vi "start async worker.vi"(8 "error in":errorcluster, 10 "run flag":u8 format="%.0b", 11 "module data in":T1={"run state"=enum."sync", "module"=refnum, "module ref"=refnum, "async exec ref"={"command fifo"=refnum, "error fifo"=refnum, "VI Refnum"=refnum, "input buffer"=refnum, "output buffer"=refnum, "process buffer"=refnum, "original dvrs"=[]}, "configuration ref"=refnum, "GUID"={"Hi"=0, "Lo"=0}, "error"={"status"=FALSE, "code"=0, "source"=""}, "previous error code"=0, "input method"={"data table"={"Double"=[], "Single"=[], "I64"=[], "I32"=[], "I16"=[], "I8"=[], "U64"=[], "U32"=[], "U16"=[], "U8"=[], "Boolean"=[], "String"=[], "Array of Double"=[], "Array of Single"=[], "Array of I64"=[], "Array of I32"=[], "Array of I16"=[], "Array of I8"=[], "Array of U64"=[], "Array of U32"=[], "Array of U16"=[], "Array of U8"=[], "Array of Boolean"=[], "Array of String"=[]}, "transfer spec"=[]}, "output method"={"data table"={"Double"=[], "Single"=[], "I64"=[], "I32"=[], "I16"=[], "I8"=[], "U64"=[], "U32"=[], "U16"=[], "U8"=[], "Boolean"=[], "String"=[], "Array of Double"=[], "Array of Single"=[], "Array of I64"=[], "Array of I32"=[], "Array of I16"=[], "Array of I8"=[], "Array of U64"=[], "Array of U32"=[], "Array of U16"=[], "Array of U8"=[], "Array of Boolean"=[], "Array of String"=[]}, "transfer spec"=[]}, "process method parameters"={"data table"={"Double"=[], "Single"=[], "I64"=[], "I32"=[], "I16"=[], "I8"=[], "U64"=[], "U32"=[], "U16"=[], "U8"=[], "Boolean"=[], "String"=[], "Array of Double"=[], "Array of Single"=[], "Array of I64"=[], "Array of I32"=[], "Array of I16"=[], "Array of I8"=[], "Array of U64"=[], "Array of U32"=[], "Array of U16"=[], "Array of U8"=[], "Array of Boolean"=[], "Array of String"=[]}, "transfer spec"=[]}, "process method results"={"data table"={"Double"=[], "Single"=[], "I64"=[], "I32"=[], "I16"=[], "I8"=[], "U64"=[], "U32"=[], "U16"=[], "U8"=[], "Boolean"=[], "String"=[], "Array of Double"=[], "Array of Single"=[], "Array of I64"=[], "Array of I32"=[], "Array of I16"=[], "Array of I8"=[], "Array of U64"=[], "Array of U32"=[], "Array of U16"=[], "Array of U8"=[], "Array of Boolean"=[], "Array of String"=[]}, "transfer spec"=[]}, "fault handling"={"unknown"=[], "trivial"=[], "critical"=[], "recoverable"=[]}, "error report index "=-1} {"GUID"."Lo" format="%.0x"; "GUID"."Hi" format="%.0x"}) -> (0 "error out":errorcluster, 3 "module data out":T1={"run state"=enum."sync", "module"=refnum, "module ref"=refnum, "async exec ref"={"command fifo"=refnum, "error fifo"=refnum, "VI Refnum"=refnum, "input buffer"=refnum, "output buffer"=refnum, "process buffer"=refnum, "original dvrs"=[]}, "configuration ref"=refnum, "GUID"={"Hi"=0, "Lo"=0}, "error"={"status"=FALSE, "code"=0, "source"=""}, "previous error code"=0, "input method"={"data table"={"Double"=[], "Single"=[], "I64"=[], "I32"=[], "I16"=[], "I8"=[], "U64"=[], "U32"=[], "U16"=[], "U8"=[], "Boolean"=[], "String"=[], "Array of Double"=[], "Array of Single"=[], "Array of I64"=[], "Array of I32"=[], "Array of I16"=[], "Array of I8"=[], "Array of U64"=[], "Array of U32"=[], "Array of U16"=[], "Array of U8"=[], "Array of Boolean"=[], "Array of String"=[]}, "transfer spec"=[]}, "output method"={"data table"={"Double"=[], "Single"=[], "I64"=[], "I32"=[], "I16"=[], "I8"=[], "U64"=[], "U32"=[], "U16"=[], "U8"=[], "Boolean"=[], "String"=[], "Array of Double"=[], "Array of Single"=[], "Array of I64"=[], "Array of I32"=[], "Array of I16"=[], "Array of I8"=[], "Array of U64"=[], "Array of U32"=[], "Array of U16"=[], "Array of U8"=[], "Array of Boolean"=[], "Array of String"=[]}, "transfer spec"=[]}, "process method parameters"={"data table"={"Double"=[], "Single"=[], "I64"=[], "I32"=[], "I16"=[], "I8"=[], "U64"=[], "U32"=[], "U16"=[], "U8"=[], "Boolean"=[], "String"=[], "Array of Double"=[], "Array of Single"=[], "Array of I64"=[], "Array of I32"=[], "Array of I16"=[], "Array of I8"=[], "Array of U64"=[], "Array of U32"=[], "Array of U16"=[], "Array of U8"=[], "Array of Boolean"=[], "Array of String"=[]}, "transfer spec"=[]}, "process method results"={"data table"={"Double"=[], "Single"=[], "I64"=[], "I32"=[], "I16"=[], "I8"=[], "U64"=[], "U32"=[], "U16"=[], "U8"=[], "Boolean"=[], "String"=[], "Array of Double"=[], "Array of Single"=[], "Array of I64"=[], "Array of I32"=[], "Array of I16"=[], "Array of I8"=[], "Array of U64"=[], "Array of U32"=[], "Array of U16"=[], "Array of U8"=[], "Array of Boolean"=[], "Array of String"=[]}, "transfer spec"=[]}, "fault handling"={"unknown"=[], "trivial"=[], "critical"=[], "recoverable"=[]}, "error report index "=-1} {"GUID"."Lo" format="%.0x"; "GUID"."Hi" format="%.0x"})   [LabVIEW 2013, in "async executor.lvlib"]
uses:
  async executor.lvlib
  Runtime/full module data.ctl
  <vilib>/NI/Tag Bus Module Framework/runtime/TBM module execution interface.lvclass
  Runtime/module run state.ctl
  asynchronous executor reference.ctl
  message to executor.ctl
  Runtime/async command notification.ctl
  <vilib>/NI/Tag Bus/table/data table.ctl
  Runtime/async error info.ctl
  <vilib>/NI/Tag Bus Module Framework/runtime/error classification.ctl
  <vilib>/NI/Tag Bus Module Framework/module configuration/TBM module configuration.lvclass
  <vilib>/NI/Configuration Framework/serializable configuration/Numeric GUID.ctl
  Runtime/module method data.ctl
  <vilib>/NI/Tag Bus/table/transfer specification.ctl
  <vilib>/NI/Tag Bus/tag/Data Type.ctl
  Runtime/fault handling spec.ctl
  Configuration/Error Actions.ctl
  async worker process.vi
  <vilib>/NI/Tag Bus/table/data table.lvlib
  main engine/main engine.lvlib
  <vilib>/NI/Tag Bus/tag/tag descriptor.lvclass
  Configuration/Standard Engine Configuration.lvclass
  <vilib>/NI/Configuration Framework/serializable configuration/NISE_CEF_serializable configuration.lvclass
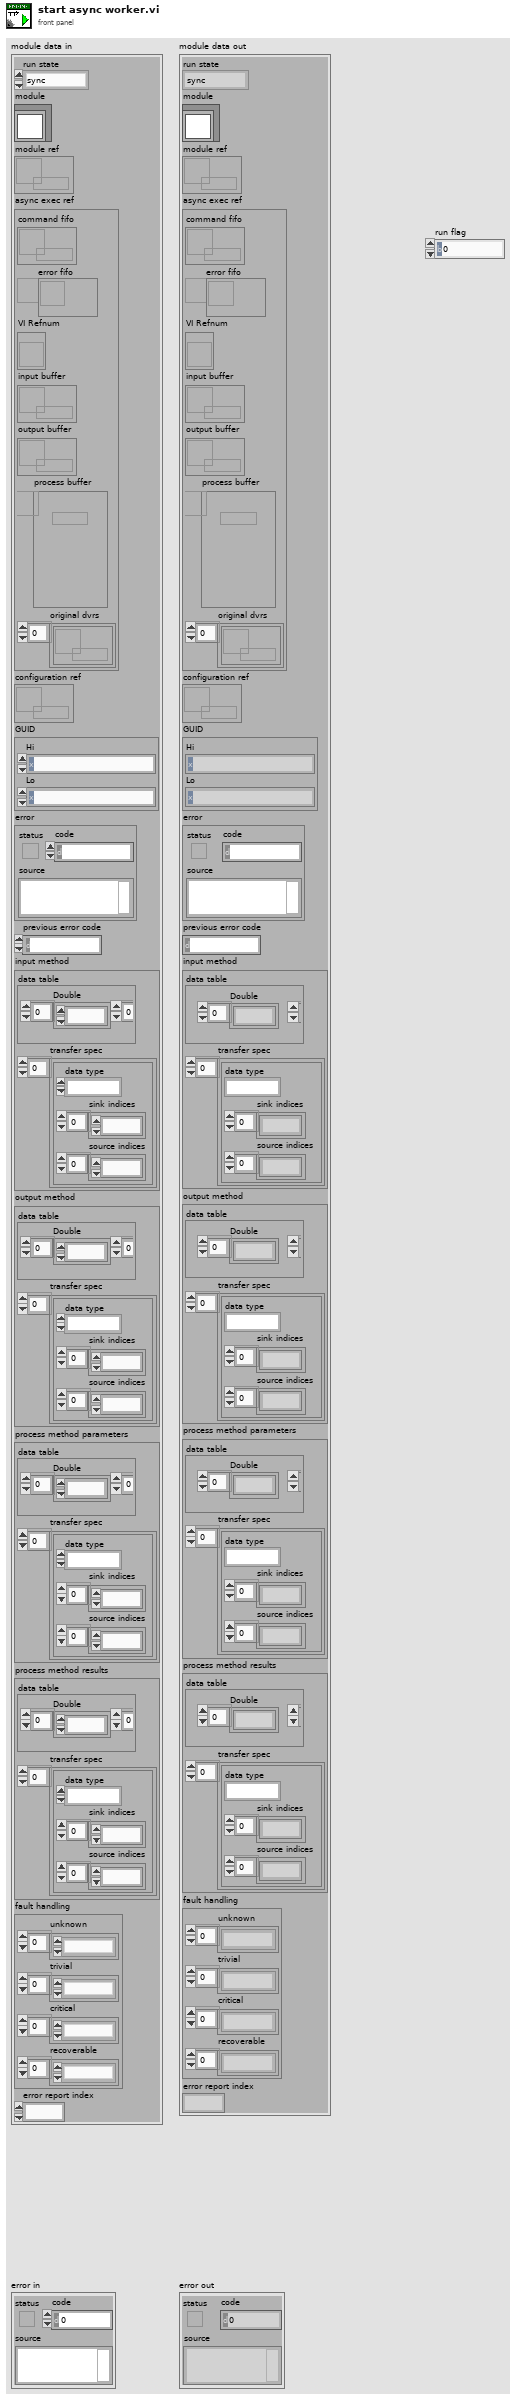
[diagram p1: front panel]
types:
  T1 = typedef "main engine.lvlib/full module data.ctl" = cluster{"run state":T2, "module":refnum<class "TBM module execution interface.lvclass">, "module ref":refnum<data-value>, "async exec ref":T3, "configuration ref":refnum<data-value>, "GUID":T4, "error":errorcluster, "previous error code":i32, "input method":T5, "output method":T5, "process method parameters":T5, "process method results":T5, "fault handling":T9, "error report index ":i32}
  T2 = typedef "main engine.lvlib/module run state.ctl" = enum16{"sync", "async"}
  T3 = typedef "async executor.lvlib/asynchronous executor reference.ctl" = cluster{"command fifo":refnum<k33>, "error fifo":refnum<k33>, "VI Refnum":refnum<vi>, "input buffer":refnum<k33>, "output buffer":refnum<k33>, "process buffer":refnum<k33>, "original dvrs":refnum<data-value>[]}
  T4 = typedef "NISE_CEF_serializable configuration.lvclass/Numeric GUID.ctl" = cluster{"Hi":u64, "Lo":u64}
  T5 = typedef "main engine.lvlib/module method data.ctl" = cluster{"data table":T6, "transfer spec":T7[]}
  T6 = typedef "tag bus.lvlib/data table.lvlib/data table.ctl" = cluster{"Double":dbl[], "Single":sgl[], "I64":i64[], "I32":i32[], "I16":i16[], "I8":i8[], "U64":u64[], "U32":u32[], "U16":u16[], "U8":u8[], "Boolean":bool[], "String":string[], "Array of Double":cluster{"DBL Array":dbl[]}[], "Array of Single":cluster{"SGL Array":sgl[]}[], "Array of I64":cluster{"I64 Array":i64[]}[], "Array of I32":cluster{"I32 Array":i32[]}[], "Array of I16":cluster{"I16 Array":i16[]}[], "Array of I8":cluster{"I8 Array":i8[]}[], "Array of U64":cluster{"U64 Array":u64[]}[], "Array of U32":cluster{"U32 Array":u32[]}[], "Array of U16":cluster{"U16 Array":u16[]}[], "Array of U8":cluster{"U8 Array":u8[]}[], "Array of Boolean":cluster{"Boolean Array":bool[]}[], "Array of String":cluster{"String Array":string[]}[]}
  T7 = typedef "tag bus.lvlib/data table.lvlib/transfer specification.ctl" = cluster{"data type":T8, "sink indices":i32[], "source indices":i32[]}
  T8 = typedef "tag bus.lvlib/tag descriptor.lvclass/Data Type.ctl" = enum16{"Double", "Single", "I64", "I32", "I16", "I8", "U64", "U32", "U16", "U8", "Boolean", "String", "Array of Double", "Array of Single", "Array of I64", "Array of I32", "Array of I16", "Array of I8", "Array of U64", "Array of U32", "Array of U16", "Array of U8", "Array of Boolean", "Array of String"}
  T9 = typedef "main engine.lvlib/fault handling spec.ctl" = cluster{"unknown":T10[], "trivial":T10[], "critical":T10[], "recoverable":T10[]}
  T10 = typedef "Standard Engine Configuration.lvclass/Error Actions.ctl" = enum16{"Clear", "Notify", "Stop Component", "Stop Engine", "Safe State", "Attempt Recovery"}
  T11 = cluster{"parameters":refnum<data-value>, "results":refnum<data-value>}
  T12 = cluster{"read mode":enum16{"polling", "blocking"}, "write mode":enum16{"polling", "blocking"}}
  T13 = typedef "async executor.lvlib/message to executor.ctl" = cluster{"command":T14, "data 1 (i,o,pp)":refnum<data-value>, "data 2 (pr)":refnum<data-value>, "user value":u64}
  T14 = typedef "async executor.lvlib/async command notification.ctl" = enum16{"stop", "input", "process", "output"}
  T15 = typedef "async executor.lvlib/async error info.ctl" = cluster{"error code":i32, "error classification":T16}
  T16 = typedef "TBM module execution interface.lvclass/error classification.ctl" = enum16{"unknown", "none", "trivial", "recoverable", "critical"}
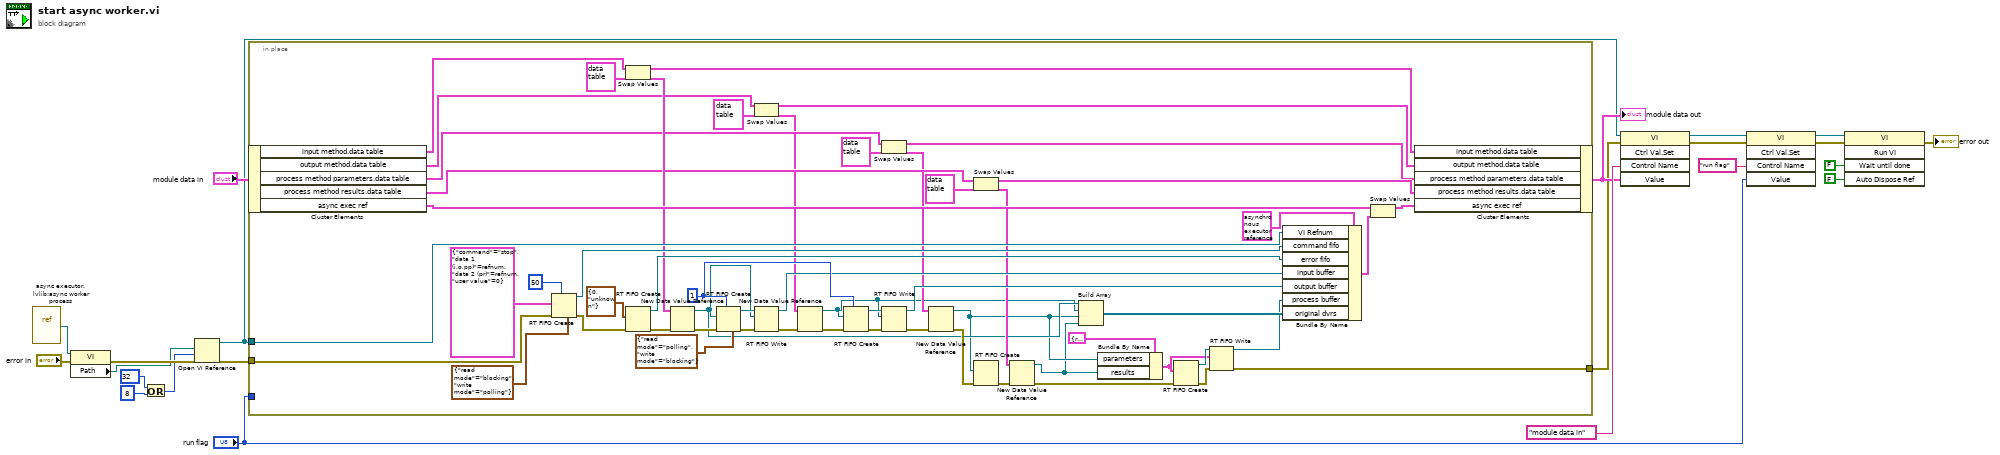
[diagram p0: block diagram]
diagram:
  n1 = vi-ref "async executor.lvlib:async worker process.vi"() -> (w20:refnum<vi>)
  n2 = property class="VI"(reference=w20, error in="error in") -> (error out=w21:errorcluster, "Path"=w19:path)  [unwired: 1 out]
  n3 = Or(x=32 ("options"), y=8 ("options")) -> (x .or. y?=w14:i32)
  n4 = Open VI Reference(vi path=w19, options=w14, error in (no error)=w21) -> (vi reference=w2:refnum<vi>, error out=w3:errorcluster)  [unwired: 3 in]
  n5 = in-place {
    in-place-border: "run flag" -> [_]
    in-place-border: w3 -> [w76]
    in-place-border: w2 -> [w75]
    in-place-border: [w50] -> w1
    w55 = u32 1 ("size (10)")
    n6 = in-place-cluster #1("module data in") -> ("input method.data table"=w42:T6, "output method.data table"=w29:T6, "process method parameters.data table"=w32:T6, "process method results.data table"=w34:T6, "async exec ref"=w56:T3)
    n7 = RT FIFO Create(1:T13 {"command"=enum."stop", "data 1 (i,o,pp)"=refnum, "data 2 (pr)"=refnum, "user value"=0} ("data to process"), 3:w76, 4:u32 50 ("size (10)"), 7:T12 {"read mode"=enum."blocking", "write mode"=enum."polling"} ("r/w modes (polling,polling)")) -> (8:w73:refnum<k33>, 11:w74:errorcluster)  [unwired: 4 in, 1 out]
    n8 = Swap Values(12:w42, 14:T6 {"Double"=[], "Single"=[], "I64"=[], "I32"=[], "I16"=[], "I8"=[], "U64"=[], "U32"=[], "U16"=[], "U8"=[], "Boolean"=[], "String"=[], "Array of Double"=[], "Array of Single"=[], "Array of I64"=[], "Array of I32"=[], "Array of I16"=[], "Array of I8"=[], "Array of U64"=[], "Array of U32"=[], "Array of U16"=[], "Array of U8"=[], "Array of Boolean"=[], "Array of String"=[]} ("y'")) -> (1:w41:T6, 3:w39:T6)  [unwired: 1 in]
    n9 = RT FIFO Create(1:T15 {"error code"=0, "error classification"=enum."unknown"} ("error information"), 3:w74) -> (8:w71:refnum<k33>, 11:w54:errorcluster)  [unwired: 6 in, 1 out]
    n10 = New Data Value Reference(data value=w39, error in=w54) -> (data value reference=w26:refnum<data-value>, error out=w69:errorcluster)
    n11 = RT FIFO Create(1:w26, 3:w69, 4:w55, 7:T12 {"read mode"=enum."polling", "write mode"=enum."blocking"} ("r/w modes (polling,polling)")) -> (8:w67:refnum<k33>, 11:w68:errorcluster)  [unwired: 4 in, 1 out]
    n12 = Swap Values(12:w29, 14:T6 {"Double"=[], "Single"=[], "I64"=[], "I32"=[], "I16"=[], "I8"=[], "U64"=[], "U32"=[], "U16"=[], "U8"=[], "Boolean"=[], "String"=[], "Array of Double"=[], "Array of Single"=[], "Array of I64"=[], "Array of I32"=[], "Array of I16"=[], "Array of I8"=[], "Array of U64"=[], "Array of U32"=[], "Array of U16"=[], "Array of U8"=[], "Array of Boolean"=[], "Array of String"=[]} ("y'")) -> (1:w27:T6, 3:w28:T6)  [unwired: 1 in]
    n13 = RT FIFO Write(0:w67, 1:w26, 3:w68) -> (8:w48:refnum<k33>, 11:w53:errorcluster)  [unwired: 2 in, 2 out]
    n14 = New Data Value Reference(data value=w28, error in=w53) -> (data value reference=w25:refnum<data-value>, error out=w61:errorcluster)
    n15 = RT FIFO Create(1:w25, 3:w61, 4:w55) -> (8:w63:refnum<k33>, 11:w62:errorcluster)  [unwired: 5 in, 1 out]
    n16 = Swap Values(12:w32, 14:T6 {"Double"=[], "Single"=[], "I64"=[], "I32"=[], "I16"=[], "I8"=[], "U64"=[], "U32"=[], "U16"=[], "U8"=[], "Boolean"=[], "String"=[], "Array of Double"=[], "Array of Single"=[], "Array of I64"=[], "Array of I32"=[], "Array of I16"=[], "Array of I8"=[], "Array of U64"=[], "Array of U32"=[], "Array of U16"=[], "Array of U8"=[], "Array of Boolean"=[], "Array of String"=[]} ("y'")) -> (1:w31:T6, 3:w30:T6)  [unwired: 1 in]
    n17 = RT FIFO Write(0:w63, 1:w25, 3:w62) -> (8:w49:refnum<k33>, 11:w52:errorcluster)  [unwired: 2 in, 2 out]
    n18 = New Data Value Reference(data value=w30, error in=w52) -> (data value reference=w24:refnum<data-value>, error out=w60:errorcluster)
    n19 = Swap Values(12:w34, 14:T6 {"Double"=[], "Single"=[], "I64"=[], "I32"=[], "I16"=[], "I8"=[], "U64"=[], "U32"=[], "U16"=[], "U8"=[], "Boolean"=[], "String"=[], "Array of Double"=[], "Array of Single"=[], "Array of I64"=[], "Array of I32"=[], "Array of I16"=[], "Array of I8"=[], "Array of U64"=[], "Array of U32"=[], "Array of U16"=[], "Array of U8"=[], "Array of Boolean"=[], "Array of String"=[]} ("y'")) -> (1:w33:T6, 3:w35:T6)  [unwired: 1 in]
    n20 = RT FIFO Create(1:w24, 3:w60) -> (11:w51:errorcluster)  [unwired: 6 in, 2 out]
    n21 = New Data Value Reference(data value=w35, error in=w51) -> (data value reference=w23:refnum<data-value>, error out=w57:errorcluster)
    n22 = Build Array(w26, w25, w24, w23) -> (w46:refnum<data-value>[])
    n23 = Bundle By Name(cluster=T11 {"parameters"=refnum, "results"=refnum} ("process data"), "parameters"=w24, "results"=w23) -> (w44:T11)
    n24 = RT FIFO Create(1:w44, 3:w57) -> (8:w59:refnum<k33>, 11:w58:errorcluster)  [unwired: 6 in, 1 out]
    n25 = RT FIFO Write(0:w59, 1:w44, 3:w58) -> (8:w43:refnum<k33>, 11:w50:errorcluster)  [unwired: 2 in, 2 out]
    n26 = Bundle By Name(cluster=T3 {"command fifo"=refnum, "error fifo"=refnum, "VI Refnum"=refnum, "input buffer"=refnum, "output buffer"=refnum, "process buffer"=refnum, "original dvrs"=[]} ("async exec ref"), "VI Refnum"=w75, "command fifo"=w73, "error fifo"=w71, "input buffer"=w48, "output buffer"=w49, "process buffer"=w43, "original dvrs"=w46) -> (w77:T3)
    n27 = Swap Values(12:w56, 14:w77) -> (1:w70:T3)  [unwired: 1 in, 1 out]
    n28 = in-place-cluster #1("input method.data table"=w41, "output method.data table"=w27, "process method parameters.data table"=w31, "process method results.data table"=w33, "async exec ref"=w70) -> (w5:T1)
  }
  "module data out" <- w5
  n29 = invoke class="VI" method="Ctrl Val.Set"(reference=w2, error in=w1, "Control Name"="module data in", "Value"=w5) -> (reference out=w8:refnum<vi>, error out=w12:errorcluster)  [unwired: 1 in, 3 out]
  n30 = invoke class="VI" method="Ctrl Val.Set"(reference=w8, error in=w12, "Control Name"="run flag", "Value"="run flag") -> (reference out=w7:refnum<vi>, error out=w9:errorcluster)  [unwired: 1 in, 3 out]
  n31 = invoke class="VI" method="Run VI"(reference=w7, error in=w9, "Wait until done"=FALSE ("Wait Until Done"), "Auto Dispose Ref"=FALSE ("Auto Dispose Reference")) -> (error out=→"error out":errorcluster)  [unwired: 1 in, 4 out]
